vi "QSM LV2.vi"(0 "Queue Name":string, 5 "Enqueue N":string[](array[string]), 9 "Enqueue? (T)":bool=TRUE, 11 "Error In":errorcluster, 12 "Command":T1=enum."Enqueue N") -> (4 "Dequeue":string, 15 "Error Out":errorcluster)   [LabVIEW 2014, in "Dragon Tamers.lvlib"]
uses:
  Dragon Tamers.lvlib
  Typedefs/Queue Commands.ctl
panel:
  in  "State In":string
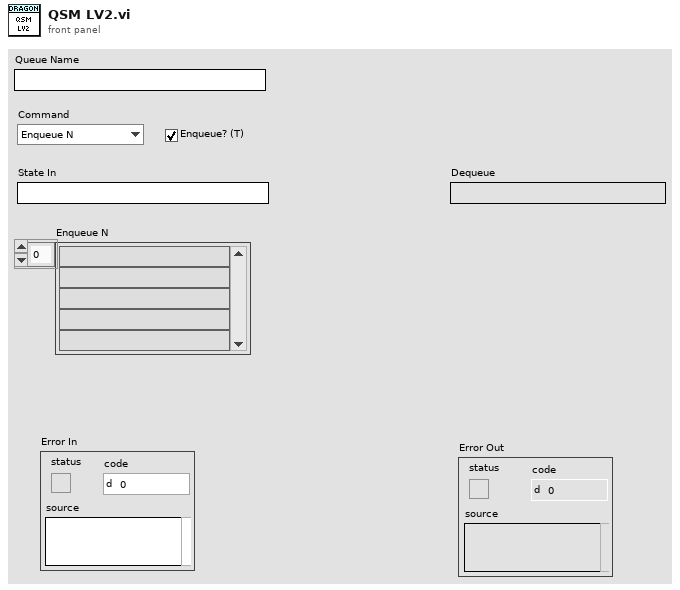
[diagram p1: front panel]
types:
  T1 = typedef "Dragon Tamers.lvlib/Queue Commands.ctl" = enum16{"Create", "Enqueue", "Enqueue N", "Enstack", "Dequeue", "Flush", "Release"}
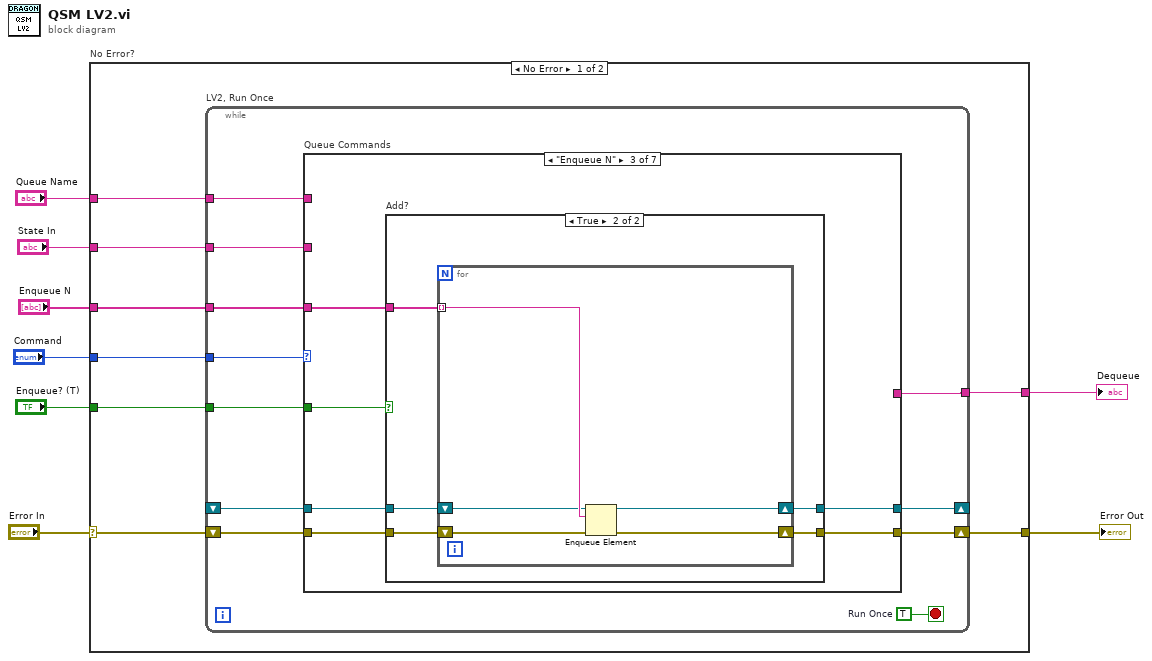
[diagram p0: block diagram]
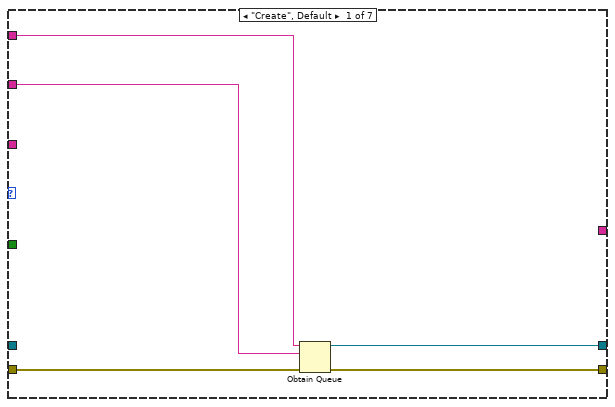
[diagram p2: hidden frame]
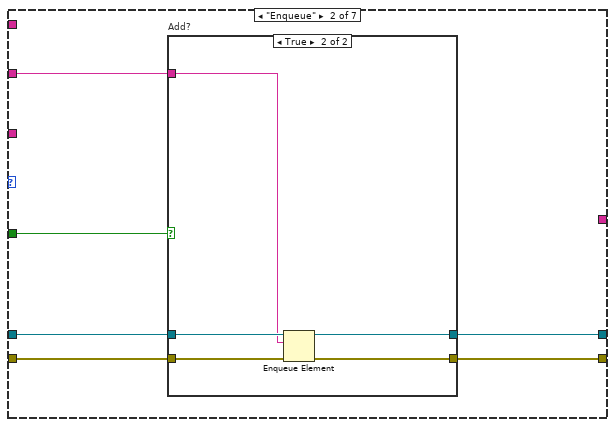
[diagram p3: hidden frame]
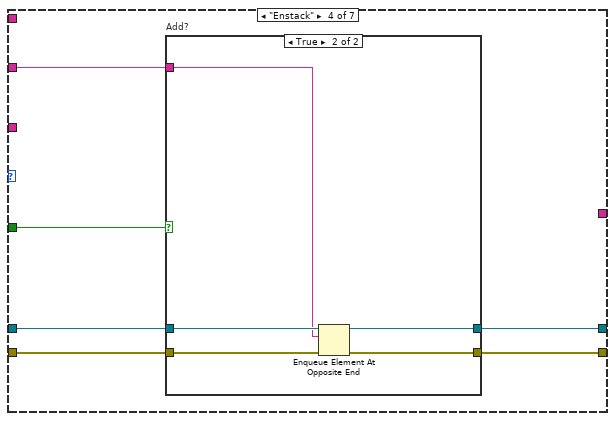
[diagram p6: hidden frame]
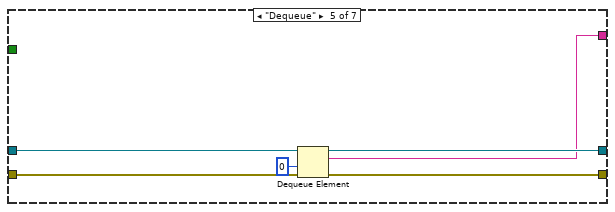
[diagram p8: hidden frame]
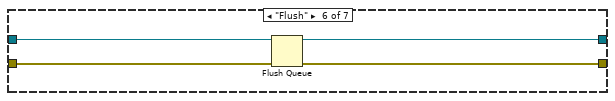
[diagram p9: hidden frame]
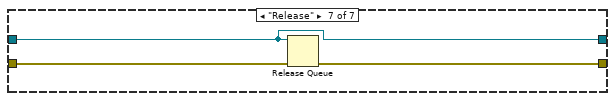
[diagram p10: hidden frame]
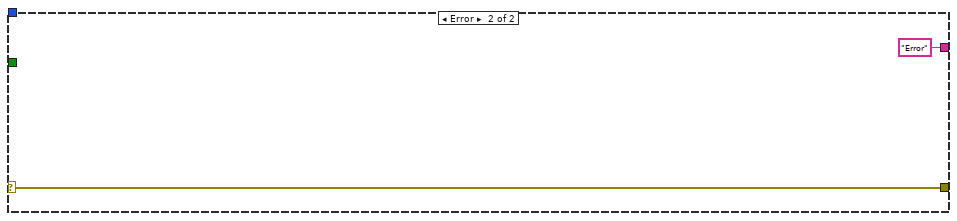
[diagram p11: hidden frame]
diagram:
  n1 = case "No Error?" shown="No Error" "Error In" {
    selector: "Error In" -> [w10 w91]
    tunnel: "Command" -> [w16 _]
    tunnel: [w15 w91] -> w7
    tunnel: "Queue Name" -> [w14 _]
    tunnel: "State In" -> [w13 _]
    tunnel: "Enqueue N" -> [w12 _]
    tunnel: [w11 "Error" ("State In")] -> w3
    tunnel: "Enqueue? (T)" -> [w9 _]
    frame No Error {
      n2 = while "LV2, Run Once" {
        tunnel: w16 -> [w26]
        shift-right: [w24] -> w15
        shift-left: w10 -> [w25]
        tunnel: w14 -> [w23]
        tunnel: w13 -> [w22]
        shift-right: [w21] -> _
        shift-left: _ -> [w20]
        tunnel: w12 -> [w19]
        tunnel: [w18] -> w11
        tunnel: w9 -> [w17]
        stop <- w27 stop-if-true
        w27 = TRUE  # Run Once
        n3 = case "Queue Commands" shown="\"Enqueue N\"" w26 {
          tunnel: w25 -> [w32 w36 w51 w69 w82 w86 w89]
          tunnel: [w31 w35 w50 w68 w81 w85 w88] -> w24
          tunnel: w23 -> [w30 _ _ _ _ _ _]
          tunnel: w22 -> [w29 w34 _ w65 _ _ _]
          tunnel: [w28 w37 w47 w66 w79 w83 w87] -> w21
          tunnel: w20 -> [_ w38 w48 w67 w80 w84 w87]
          tunnel: w19 -> [_ _ w49 _ _ _ _]
          tunnel: [_ _ _ _ w78 _ _] -> w18
          tunnel: w17 -> [_ w33 w46 w64 _ _ _]
          frame "Create", Default {
            n4 = Obtain Queue(name (unnamed)=w30, element data type=w29, error in (no error)=w32) -> (queue out=w28:refnum<queue>, error out=w31:errorcluster)  [unwired: 2 in, 1 out]
          }
          frame "Enqueue" {
            n5 = case "Add?" shown="True" w33 {
              tunnel: w38 -> [w40 w45]
              tunnel: [w40 w44] -> w37
              tunnel: w36 -> [w39 w43]
              tunnel: [w39 w42] -> w35
              tunnel: w34 -> [_ w41]
              frame False {
              }
              frame True {
                n6 = Enqueue Element(queue=w45, element=w41, error in (no error)=w43) -> (queue out=w44:refnum<queue>, error out=w42:errorcluster)  [unwired: 1 in, 1 out]
              }
            }
          }
          frame "Enqueue N" {
            n7 = case "Add?" shown="True" w46 {
              tunnel: w51 -> [w52 w58]
              tunnel: [w52 w57] -> w50
              tunnel: w49 -> [_ w56]
              tunnel: w48 -> [w53 w55]
              tunnel: [w53 w54] -> w47
              frame False {
              }
              frame True {
                n8 = for {
                  shift-right: [w62] -> w57
                  shift-left: w58 -> [w63]
                  tunnel: w56 -> [w61] mode=indexing
                  shift-right: [w59] -> w54
                  shift-left: w55 -> [w60]
                  n9 = Enqueue Element(queue=w60, element=w61, error in (no error)=w63) -> (queue out=w59:refnum<queue>, error out=w62:errorcluster)  [unwired: 1 in, 1 out]
                }
              }
            }
          }
          frame "Enstack" {
            n10 = case "Add?" shown="True" w64 {
              tunnel: w69 -> [w70 w76]
              tunnel: [w70 w75] -> w68
              tunnel: w67 -> [w71 w74]
              tunnel: [w71 w73] -> w66
              tunnel: w65 -> [_ w72]
              frame False {
              }
              frame True {
                n11 = Enqueue Element At Opposite End(queue=w74, element=w72, error in (no error)=w76) -> (queue out=w73:refnum<queue>, error out=w75:errorcluster)  [unwired: 1 in, 1 out]
              }
            }
          }
          frame "Dequeue" {
            n12 = Dequeue Element(queue=w80, timeout in ms (-1)=0, error in (no error)=w82) -> (queue out=w79:refnum<queue>, element=w78:string, error out=w81:errorcluster)  [unwired: 1 out]
          }
          frame "Flush" {
            n13 = Flush Queue(queue=w84, error in (no error)=w86) -> (queue out=w83:refnum<queue>, error out=w85:errorcluster)  [unwired: 1 out]
          }
          frame "Release" {
            n14 = Release Queue(queue=w87, error in (no error)=w89) -> (error out=w88:errorcluster)  [unwired: 1 in, 2 out]
          }
        }
      }
    }
    frame Error {
    }
  }
  "Dequeue" <- w3
  "Error Out" <- w7
